vi "SubVI_Res_Cal.vi"(11 "Q_data":T2) -> (0 "Max Resistor":T3, 1 "PassFail":bool[](array[boolean]), 2 "Result Table update":T4, 3 "Resister result data":T5)   [LabVIEW 2016]
uses:
  Ctrls/raw data type.ctl
  Ctrls/raw Q data.ctl
  Ctrls/Fail flags.ctl
panel:
  out "Test Stop?":T1
  out "숫자형":i32
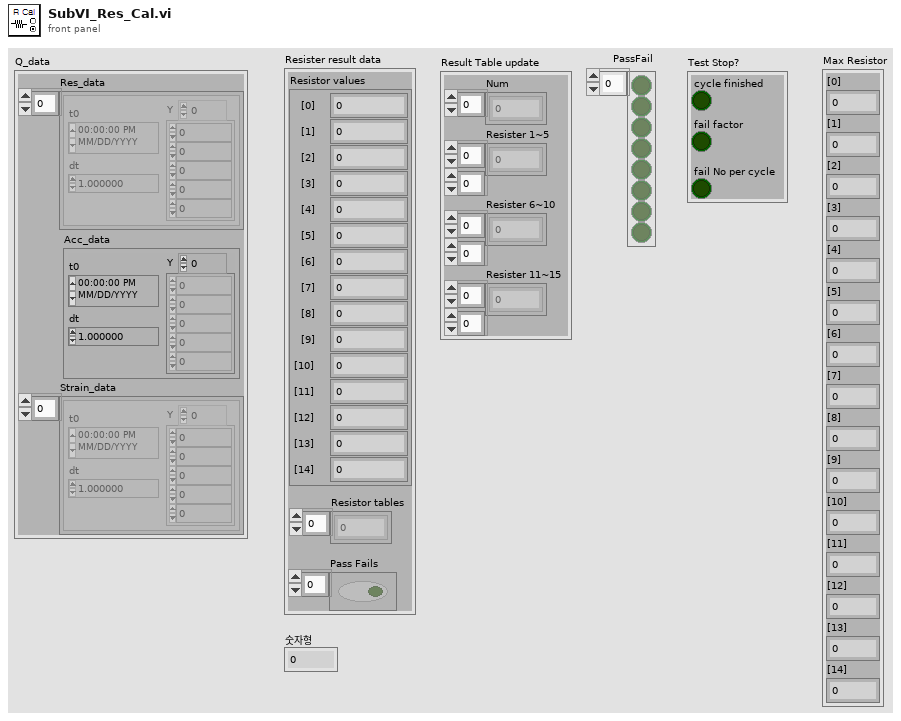
[diagram p1: front panel]
types:
  T1 = typedef "Fail flags.ctl" = cluster{"cycle finished":bool, "fail factor":bool, "fail No per cycle":bool}
  T2 = typedef "raw Q data.ctl" = cluster{"Res_data":waveform(dbl)[], "Acc_data":waveform(dbl), "Strain_data":waveform(dbl)[]}
  T3 = cluster{"[0]":dbl, "[1]":dbl, "[2]":dbl, "[3]":dbl, "[4]":dbl, "[5]":dbl, "[6]":dbl, "[7]":dbl, "[8]":dbl, "[9]":dbl, "[10]":dbl, "[11]":dbl, "[12]":dbl, "[13]":dbl, "[14]":dbl}
  T4 = cluster{"Num":u32[], "Resister 1~5":u8[][], "Resister 6~10":u8[][], "Resister 11~15":u8[][]}
  T5 = typedef "raw data type.ctl" = cluster{"Resistor values":cluster{"[0]":dbl, "[1]":dbl, "[2]":dbl, "[3]":dbl, "[4]":dbl, "[5]":dbl, "[6]":dbl, "[7]":dbl, "[8]":dbl, "[9]":dbl, "[10]":dbl, "[11]":dbl, "[12]":dbl, "[13]":dbl, "[14]":dbl}, "Resistor tables":u8[], "Pass Fails":bool[]}
  T6 = cluster{"Test Information":cluster{"date":string, "custom":string, "oper":string, "package":string, "pkg side":string, "solder":string, "brd side":string, "paste":string, "reflow":string}, "Sensor Set":cluster{"Accelerometer":cluster{"Sensitivity(mV/g)":dbl}, "Strain Guage":cluster{"Ch.":dbl[], "Gage factor":dbl[], "Resistance":dbl[], "Poisson ratio":dbl[]}}, "Resistor Set":cluster{"Criterion Level":dbl, "Res. Set":cluster{"Res. Ch":dbl, "Res. Active":bool, "Res Initial":dbl}[]}, "Test Stop Condition":cluster{"Test cycle":u16, "Fail number in a cycle":u16, "Fail factor":cluster{"Duration":u16, "Fail No.":u16}}, "Acceleration Condition ":cluster{"Shock duration pecent [%]":u16, "Filter cutoff freq":u32}, "Save":cluster{"Save Path":path, "File Name":string}}
  T7 = cluster{"Res. Ch":dbl, "Res. Active":bool, "Res Initial":dbl}[]
  T8 = typedef "Total data.ctl" = cluster{"Raw Data":T2, "Resister result data":T5, "Result Table update":cluster{"Num":u32[], "Resister 1~5":u8[][], "Resister 6~10":u8[][], "Resister 11~15":u8[][]}, "Strain Data":cluster{"Strain 1":dbl, "Strain 2":dbl, "Strain 3":dbl, "Strain 4":dbl}, "Acc Result":cluster{"Acc Peak":dbl, "Acc time":dbl, "Acc area":dbl}, "STATUS":cluster{"status":string, "all_fail":bool, "emg":bool, "cycle":u16, "file name":string}, "Speed":dbl, "Acc peak time":dbl, "Max Strain":dbl, "Resistor at peak":cluster{"[0]":dbl, "[1]":dbl, "[2]":dbl, "[3]":dbl, "[4]":dbl, "[5]":dbl, "[6]":dbl, "[7]":dbl, "[8]":dbl, "[9]":dbl, "[10]":dbl, "[11]":dbl, "[12]":dbl, "[13]":dbl, "[14]":dbl}, "Acc peak index":u32, "time":string, "Cycle finish":bool, "Resistor at ini":cluster{"[0]":dbl, "[1]":dbl, "[2]":dbl, "[3]":dbl, "[4]":dbl, "[5]":dbl, "[6]":dbl, "[7]":dbl, "[8]":dbl, "[9]":dbl, "[10]":dbl, "[11]":dbl, "[12]":dbl, "[13]":dbl, "[14]":dbl}}
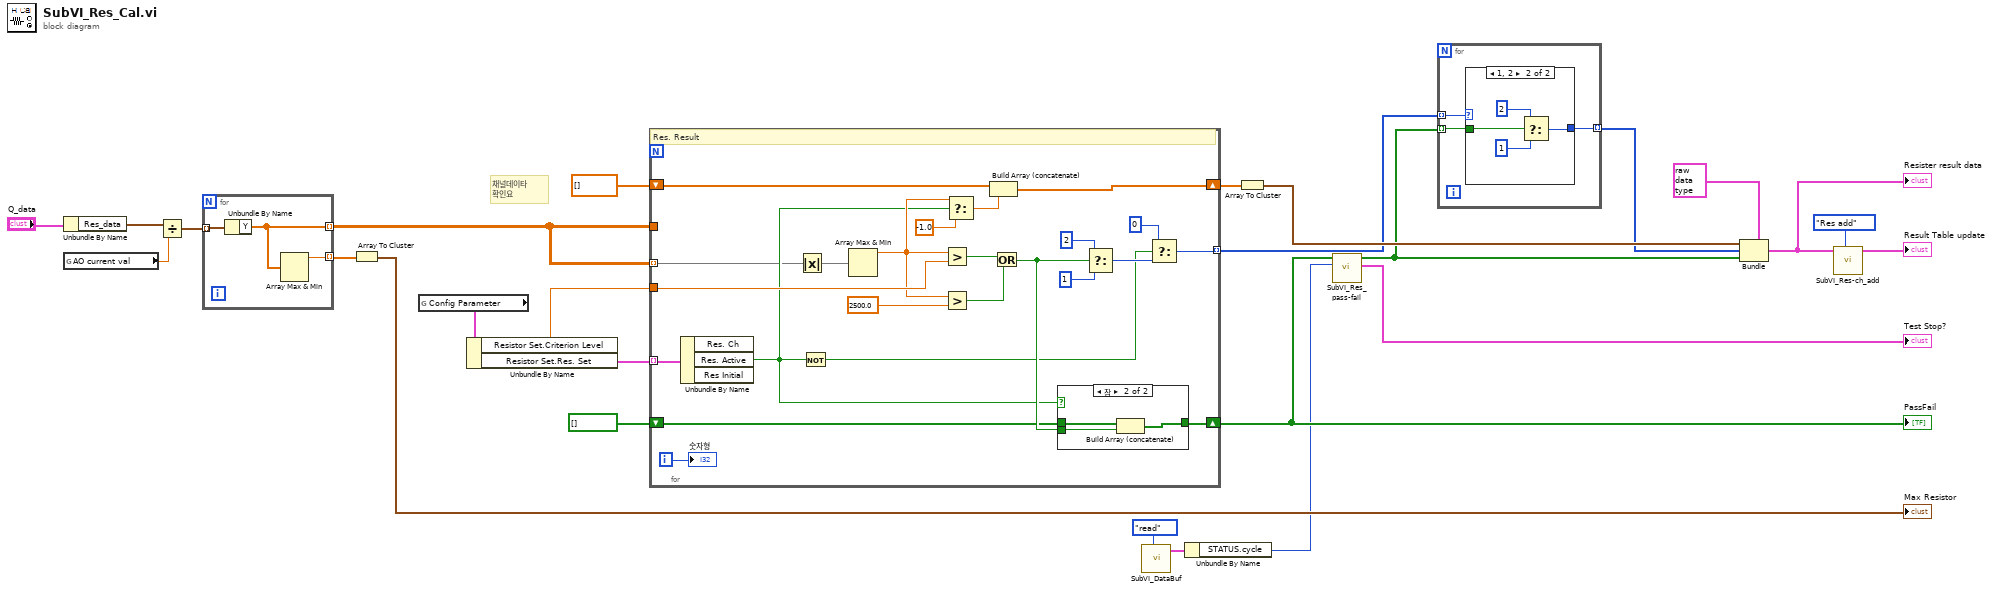
[diagram p0: block diagram]
diagram:
  # "채널데이타\n확인요"
  n1 = Unbundle By Name("Q_data") -> ("Res_data"=w15:waveform(dbl)[])
  n2 = global read "글로벌_Config Parameter.vi" "AO current val"() -> (w13:dbl)
  n3 = Divide(x=w15, y=w13) -> (x/y=w14:waveform(dbl)[])
  n4 = for {
    tunnel: w14 -> [w29] mode=indexing
    tunnel: [w28] -> w11 mode=indexing
    tunnel: [w27] -> w10 mode=indexing
    n5 = Unbundle By Name(w29) -> ("Y"=w28:dbl[])
    n6 = Array Max & Min(array=w28) -> (max value=w27:dbl)  [unwired: 3 out]
  }
  n7 = Array To Cluster(array=w10) -> (cluster=→"Max Resistor":T3)
  n8 = global read "글로벌_Config Parameter.vi" "Config Parameter"() -> (w23:T6)
  n9 = Unbundle By Name(w23) -> ("Resistor Set.Criterion Level"=w22:dbl, "Resistor Set.Res. Set"=w21:T7)
  n10 = for {
    tunnel: w21 -> [w52] mode=indexing
    shift-right: [w40] -> w8
    shift-left: bool[] [] -> [w39]
    tunnel: w11 -> [_]
    tunnel: w22 -> [w47]
    tunnel: [w42] -> w5 mode=indexing
    shift-right: [w37] -> w26
    shift-left: dbl[] [] -> [w38]
    tunnel: w11 -> [w31] mode=indexing
    i -> [w32]
    # "Res. Result"
    n11 = Unbundle By Name(w52) -> ("Res. Active"=w34:bool)  [unwired: 2 out]
    n12 = Absolute Value(x=w31) -> (abs(x)=w48:dbl[])
    n13 = Not(x=w34) -> (.not. x?=w30:bool)
    n14 = Array Max & Min(array=w48) -> (max value=w35:dbl)  [unwired: 3 out]
    n15 = Greater?(x=w35, y=w47) -> (0:w50:bool)
    n16 = Greater?(x=w35, y=2500.0) -> (0:w49:bool)
    n17 = Select(t=w35, s=w34, f=-1.0) -> (s? t:f=w36:dbl)
    n18 = Build Array (concatenate)(w38, w36) -> (w37:dbl[])
    n19 = Or(x=w50, y=w49) -> (x .or. y?=w41:bool)
    n20 = case shown="참" w34 {
      tunnel: [w53 w56] -> w40
      tunnel: w41 -> [_ w55]
      tunnel: w39 -> [w53 w54]
      frame False {
      }
      frame True {
        # "ÁÝÐ´ DÌ± ÈmÕ ÓÈ"
        n21 = Build Array (concatenate)(w54, w55) -> (w56:bool[])
      }
    }
    n22 = Select(t=u8 2, s=w41, f=u8 1) -> (s? t:f=w43:u8)
    n23 = Select(t=u8 0, s=w30, f=w43) -> (s? t:f=w42:u8)
    "숫자형" <- w32
  }
  "PassFail" <- w8
  n24 = call "SubVI_DataBuf.vi"("cmd"=enum16{"ini", "write", "read"}."read") -> ("Total data 2"=w2:T8)  [unwired: 9 in, 1 out]
  n25 = Unbundle By Name(w2) -> ("STATUS.cycle"=w1:u16)
  n26 = Array To Cluster(array=w26) -> (cluster=w20:T3)
  n27 = call "SubVI_Res_pass-fail.vi"("Current Cycle"=w1, "pass/fail"=w8) -> ("Test Stop?"=→"Test Stop?":T1, "Fail array"=w6:bool[])  [unwired: 8 in]
  n28 = for {
    tunnel: w5 -> [w59] mode=indexing
    tunnel: w6 -> [w58] mode=indexing
    tunnel: [w57] -> w4 mode=indexing
    n29 = case shown="1, 2" w59 {
      selector: w59 -> [w60 _]
      tunnel: w58 -> [_ w62]
      tunnel: [w60 w61] -> w57
      frame 0, Default {
      }
      frame 1, 2 {
        n30 = Select(t=u8 2, s=w62, f=u8 1) -> (s? t:f=w61:u8)
      }
    }
  }
  n31 = Bundle(cluster=T5 {"Resistor values"={"[0]"=0.0, "[1]"=0.0, "[2]"=0.0, "[3]"=0.0, "[4]"=0.0, "[5]"=0.0, "[6]"=0.0, "[7]"=0.0, "[8]"=0.0, "[9]"=0.0, "[10]"=0.0, "[11]"=0.0, "[12]"=0.0, "[13]"=0.0, "[14]"=0.0}, "Resistor tables"=[], "Pass Fails"=[]} ("Resister result data"), "Resistor values"=w20, "Resistor tables"=w4, "Pass Fails"=w6) -> (w17:T5)
  "Resister result data" <- w17
  n32 = call "SubVI_Res-ch_add.vi"("cmd"=enum16{"ini", "Res add", "read"}."Res add", "Resister data"=w17) -> ("Result Table update"=→"Result Table update":T4)  [unwired: 8 in, 1 out]
